vi "SP Read Array.vi"(8 "error in":errorcluster, 11 "Setpoint.lvclass":refnum<class "Setpoint.lvclass">) -> (0 "error out":errorcluster, 1 "Changed or First Call?":bool, 2 "Current Setpoint":dbl[](array[numeric]), 3 "Setpoint.lvclass 2":refnum<class "Setpoint.lvclass">)   [LabVIEW 2023, in "Setpoint.lvclass"]
uses:
  Setpoint.lvclass
  Setpoint.lvclass/Setpoint.ctl
  <vilib>/ADAS Replay HIL/Channels/Tag Wrapper/Polymorphic/Read Channel (Double).vi
  3a5e14bb-e2d6-40bb-a8f1-774026738da1.vi
  <vilib>/ADAS Replay HIL/Channels/Tag Wrapper/Polymorphic/Read Channel (Double).vi/b2f764de-0c1e-4784-a155-687fc995a684.vi
  <vilib>/ADAS Replay HIL/Channels/Tag Wrapper/Polymorphic/Read Channel (Double).vi/b2f764de-0c1e-4784-a155-687fc995a684.vi/c28b0ead-42ad-4072-80a2-aca7f2bd7ce3.vi
  <vilib>/ADAS Replay HIL/Channels/Tag Wrapper/Polymorphic/Read Channel (Double).vi/b2f764de-0c1e-4784-a155-687fc995a684.vi/219d0231-d98b-4193-b5cc-84f90e3c9091.vi
  <vilib>/ADAS Replay HIL/Channels/Tag Wrapper/Tag Wrapper.lvlib
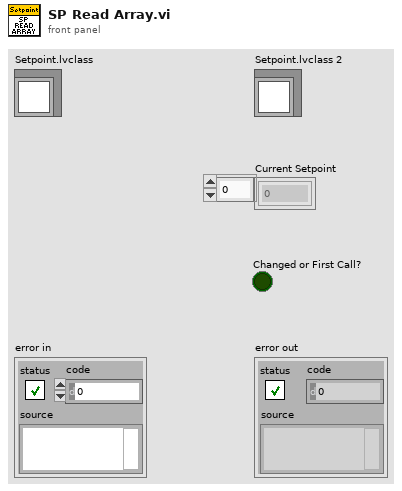
[diagram p1: front panel]
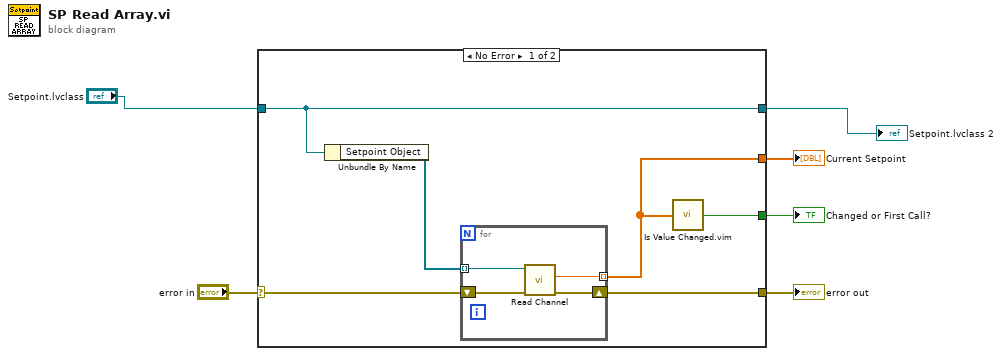
[diagram p0: block diagram]
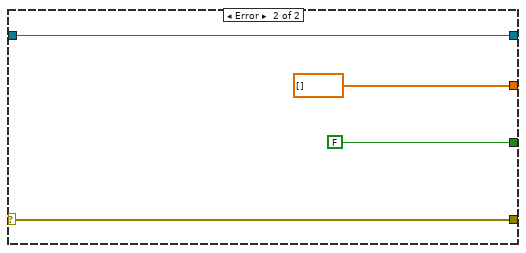
[diagram p2: hidden frame]
diagram:
  n1 = case shown="No Error" "error in" {
    selector: "error in" -> [w10 w20]
    tunnel: [w9 w20] -> w5
    tunnel: [w12 w19] -> w4
    tunnel: "Setpoint.lvclass" -> [w12 w19]
    tunnel: [w8 dbl[] []] -> w2
    tunnel: [w7 FALSE ("changed or first call?")] -> w3
    frame No Error {
      n2 = Unbundle By Name(w12) -> ("Setpoint Object"=w11:refnum<k21>[])
      n3 = for {
        tunnel: w11 -> [w16] mode=indexing
        tunnel: [w13] -> w8 mode=indexing
        shift-right: [w14] -> w9
        shift-left: w10 -> [w15]
        n4 = call-poly <vilib>:"Read Channel.vi"("error in"=w15, "ADAS HIL Channel in"=w16) -> ("error out"=w14:errorcluster, "Value out"=w13:dbl)  [unwired: 6 in, 2 out]
      }
      n5 = call "Is Value Changed.vim"("value"=w8) -> ("changed or first call?"=w7:bool)
    }
    frame Error {
    }
  }
  "error out" <- w5
  "Changed or First Call?" <- w3
  "Current Setpoint" <- w2
  "Setpoint.lvclass 2" <- w4
